vi "thermal camera.vi"() -> ()   [LabVIEW 2024]
uses:
  <vilib>/userDefined/High Color/IMAQdx.ctl
  <vilib>/vision/driver/NI_Vision_Acquisition_Software.lvlib
  irDirectSDK/examples/labview/libirimager_direct_binding.lvlib
panel:
  out "function return 3":i32
  in  "xml_config":string
  out "function return 2":i32
  out "thermal data out":u16[](array[numeric])
  out "function return":i32
  out "Image":T1(plugin-control)
  in  "stop":bool
  in  "Session In":T2
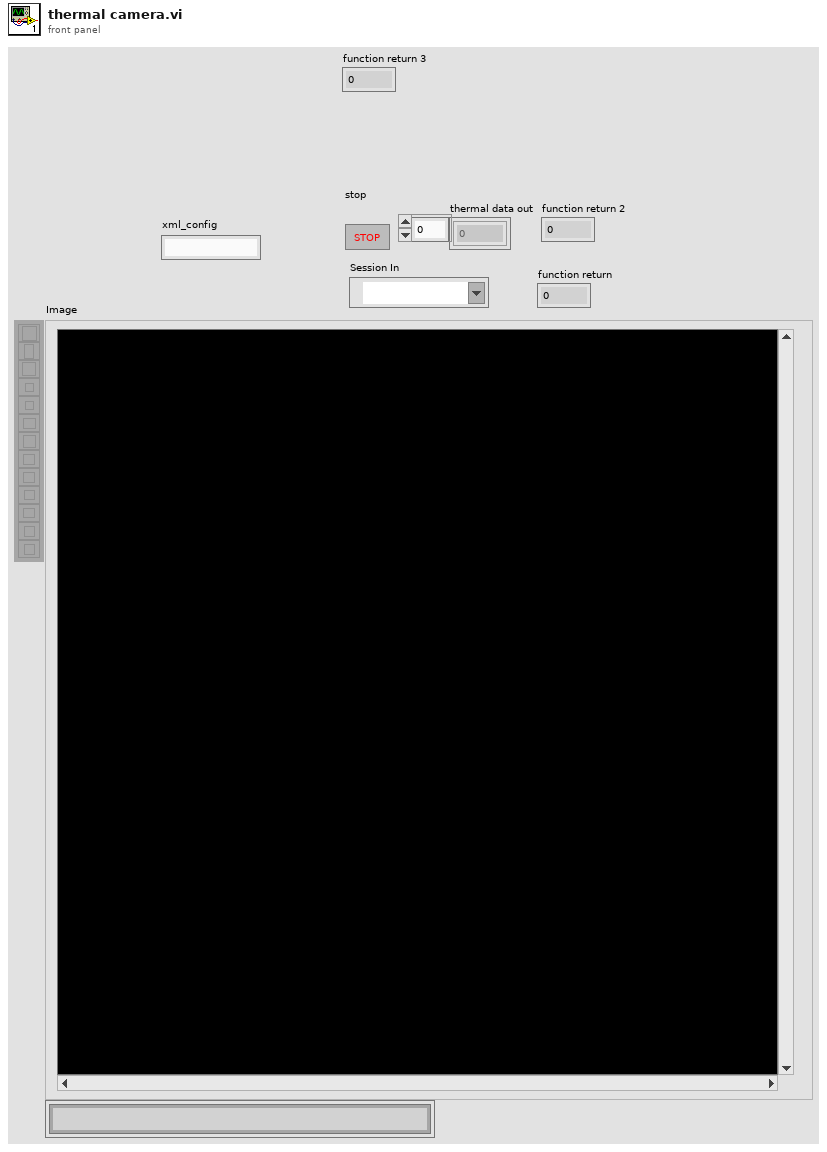
[diagram p1: front panel]
types:
  T1 = typedef "IMAQ Image.ctl" = refnum<image>
  T2 = typedef "IMAQdx.ctl" = refnum<k21>
  T3 = typedef "Image Type" = u32
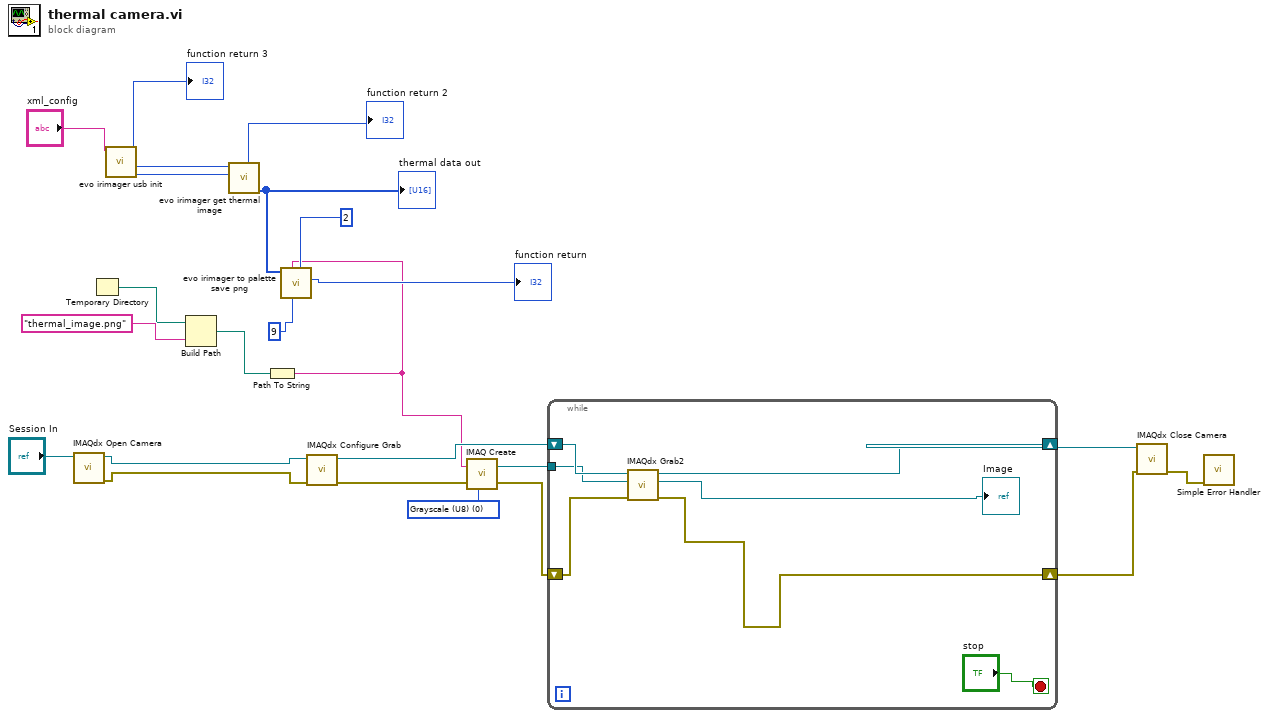
[diagram p0: block diagram]
diagram:
  w16 = T3 0 items=["Grayscale (U8)", "Grayscale (I16)", "Grayscale (SGL)", "Complex (CSG)", "RGB (U32)", "HSL (U32)", "RGB (U64)", "Grayscale (U16)"] ("Image Type")
  n1 = call <vilib>:"IMAQdx Open Camera.vi"("Session In"="Session In") -> ("error out"=w15:errorcluster, "Session Out"=w14:T2)  [unwired: 9 in]
  n2 = Temporary Directory() -> (w5:path)
  n3 = call "evo irimager usb init.vi"("xml_config"="xml_config") -> ("h out"=w3:i32, "w out"=w2:i32, "function return 2"=→"function return 3":i32)  [unwired: 7 in, 1 out]
  n4 = Build Path(base path=w5, name or relative path="thermal_image.png") -> (appended path=w7:path)
  n5 = call "evo irimager get thermal image.vi"("h"=w3, "w"=w2) -> ("data out"=w10:u16[], "function return"=→"function return 2":i32)  [unwired: 6 in, 2 out]
  "thermal data out" <- w10
  n6 = Path To String(path=w7) -> (string=w8:string)
  n7 = call "evo irimager to palette save png.vi"("palette_scale"=2, "palette"=9, "path"=w8, "thermal_data"=w10) -> ("function return"=→"function return":i32)  [unwired: 6 in, 1 out]
  n8 = call <vilib>:"IMAQdx Configure Grab.vi"("error in"=w15, "Session In"=w14) -> ("error out"=w18:errorcluster, "Session Out"=w23:T2)  [unwired: 8 in]
  n9 = call "IMAQ Create"("Image Name"=w8, "Image Type"=w16, "error in (no error)"=w18) -> ("New Image"=w20:T1, "error out"=w17:errorcluster)  [unwired: 2 in]
  n10 = while {
    shift-right: [w30] -> w22
    shift-left: w23 -> [w31]
    shift-right: [w25] -> w21
    shift-left: w17 -> [w29]
    tunnel: w20 -> [w27]
    stop <- "stop" stop-if-true
    n11 = call <vilib>:"IMAQdx Grab2.vi"("error in"=w29, "Image In"=w27, "Session In"=w31) -> ("error out"=w25:errorcluster, "Image Out"=→"Image":T1, "Session Out"=w30:T2)  [unwired: 5 in, 1 out]
  }
  n12 = call <vilib>:"IMAQdx Close Camera.vi"("error in"=w21, "Session In"=w22) -> ("error out"=w19:errorcluster)  [unwired: 9 in]
  n13 = call <vilib>:"Simple Error Handler.vi"("error in (no error)"=w19) -> ()  [unwired: 4 in, 5 out]
